vi "ShooterPrimer.vi"(0 "Left RPM":dbl, 1 "Shooter Prime":bool, 3 "Intake Mode":bool, 5 "Right RPM":dbl, 9 "Desired RPM":dbl) -> (8 "Left RPM":dbl, 12 "Left Motor Output":dbl, 14 "Right Motor Output":dbl, 15 "Right RPM":dbl)   [LabVIEW 2015]
panel:
  out "Left RPM":dbl(graph)
  out "Right RPM":dbl(graph)
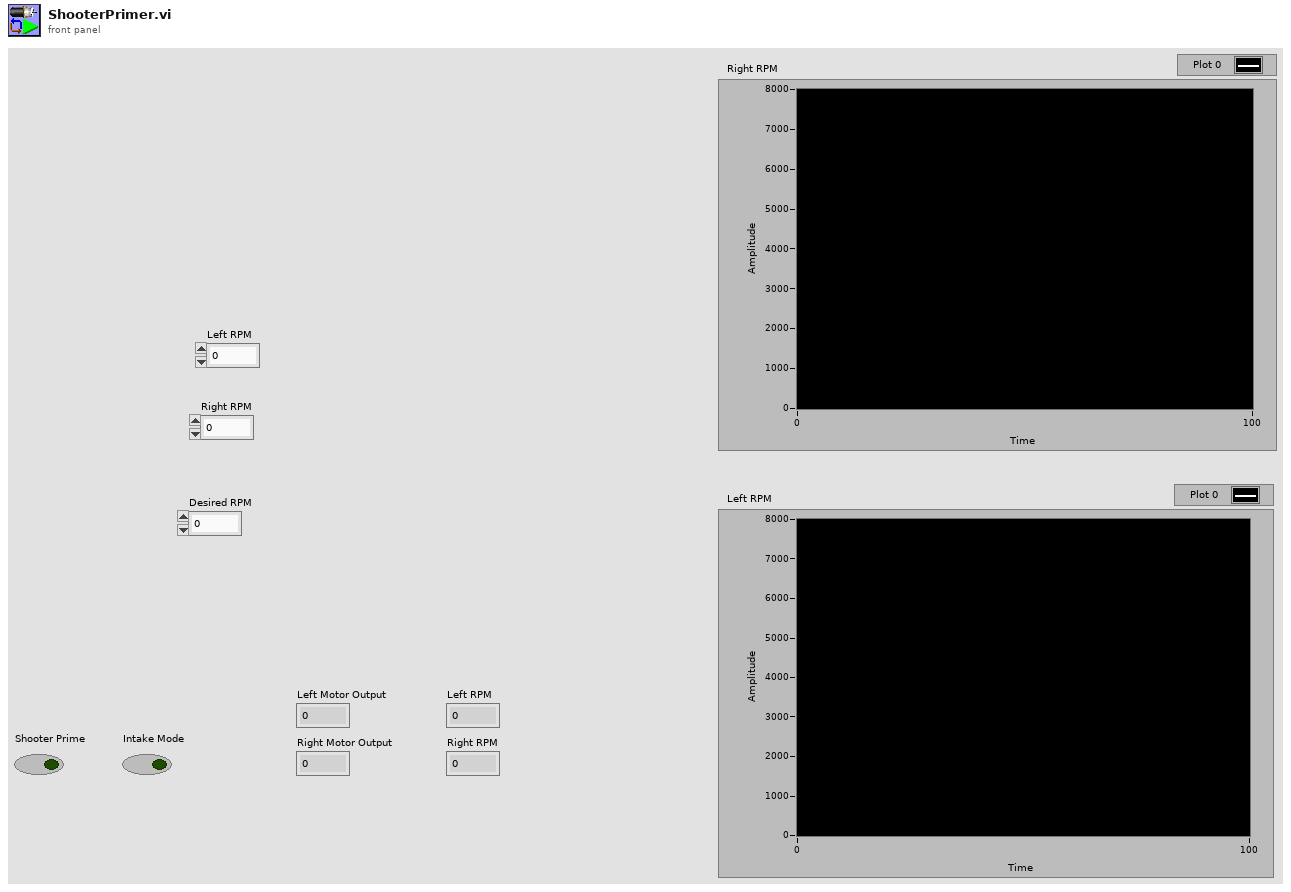
[diagram p1: front panel]
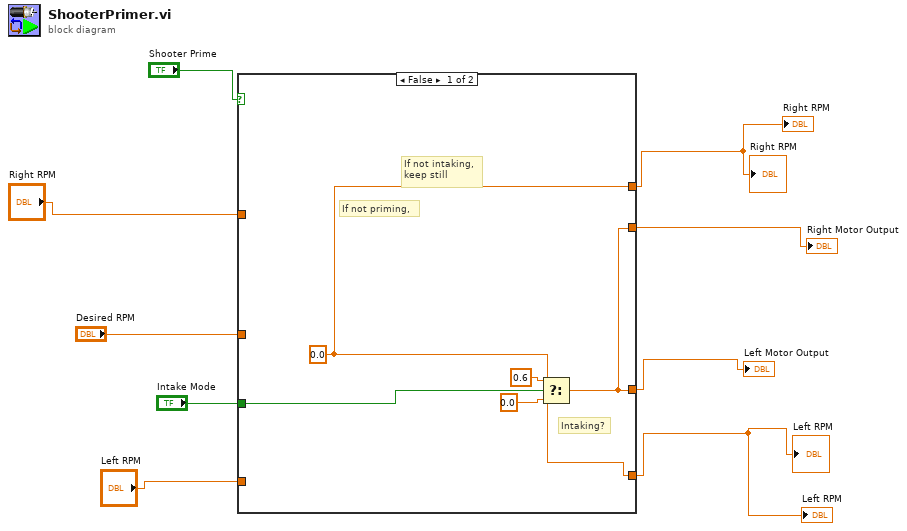
[diagram p0: block diagram]
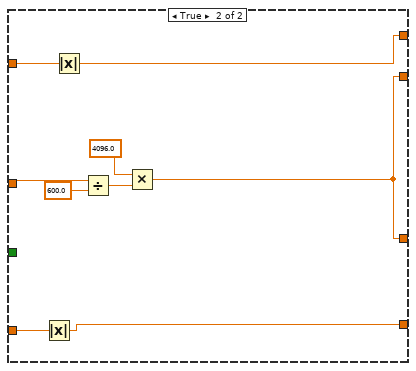
[diagram p2: hidden frame]
diagram:
  n1 = case shown="False" "Shooter Prime" {
    tunnel: [w13 w15] -> w7
    tunnel: [w13 w15] -> w6
    tunnel: "Intake Mode" -> [w11 _]
    tunnel: [w10 w20] -> w4
    tunnel: [w10 w22] -> w5
    tunnel: "Left RPM" -> [_ w23]
    tunnel: "Right RPM" -> [_ w21]
    tunnel: "Desired RPM" -> [_ w19]
    frame False {
      w10 = 0.0
      # "If not intaking,\nkeep still"
      # "Intaking?"
      # "If not priming,"
      n2 = Select(t=0.6, s=w11, f=0.0) -> (s? t:f=w13:dbl)
    }
    frame True {
      n3 = Absolute Value(x=w23) -> (abs(x)=w22:dbl)
      n4 = Absolute Value(x=w21) -> (abs(x)=w20:dbl)
      n5 = Divide(x=w19, y=600.0) -> (x/y=w17:dbl)
      n6 = Multiply(x=4096.0, y=w17) -> (x*y=w15:dbl)
    }
  }
  "Left Motor Output" <- w7
  "Right Motor Output" <- w6
  "Left RPM" <- w5
  "Right RPM" <- w4
  "Right RPM" <- w4
  "Left RPM" <- w5
